vi "Finish.vi"   [LabVIEW 2014]
doc: "This VI is called just before exiting. It is expected to close I/O refnum, save collected data, etc."
uses:
  <vilib>/Rock Robotics/WPI/Joystick/WPI_JoystickGetSetRefNum.vi
  <vilib>/Rock Robotics/WPI/RobotDrive/WPI_RobotDriveGetSetRefNum.vi
  Robot Global Data.vi
  SimpleGyro/SimpleGyro.lvlib
types:
  T1 = typedef "WPI_MotorControlDeviceRef.ctl" = cluster{"DeviceStatus":errorcluster, "Type":T2, "PWM":cluster{"Controller":T3, "PWM Channel":T4, "DeadBand":T5}, "CAN":cluster{"Device Number":u8, "Control Mode":T6, "Semaphore":T7, "Max Vout":dbl, "TalonSRX Control Mode":T8}, "Invert":bool, "TransformRef":T9, "InvTransformRef":T9}
  T2 = typedef "WPI_MotorControlType.ctl" = enum16{"PWM", "CAN", "CANTalonSRX"}
  T3 = typedef "FPGA_TypedefDigitalModule.ctl" = enum16{"Controller 1"}
  T4 = typedef "FPGA_DIOPWMChannel.ctl" = enum8{"PWM 0", "PWM 1", "PWM 2", "PWM 3", "PWM 4", "PWM 5", "PWM 6", "PWM 7", "PWM 8", "PWM 9", "PWM MXP 0", "PWM MXP 1", "PWM MXP 2", "PWM MXP 3", "PWM MXP 4", "PWM MXP 5", "PWM MXP 6", "PWM MXP 7", "PWM MXP 8", "PWM MXP 9", "Invalid"}
  T5 = typedef "WPI_PWMDeadband.ctl" = cluster{"Name":string, "maxPositivePwm":i32, "minPositivePwm":i32, "centerPwm":i32, "maxNegativePwm":i32, "minNegativePwm":i32, "angularRange":u16}
  T6 = typedef "WPI_CANJaguar_ControlMode.ctl" = enum8{"Percent VBus", "Current", "Speed", "Position", "Voltage"}
  T7 = typedef "Semaphore RefNum" = refnum<k1>
  T8 = typedef "WPI_CANTalonSRX_APIControlMode.ctl" = enum8{"Percent VBus", "Speed", "Position", "Slave", "Unchanged / Invalid"}
  T9 = typedef "WPI_PWMTransform_ConPane.ctl" = refnum<vi>
  T10 = typedef "WPI_EncoderDevRef.ctl" = cluster{"DevStatus":errorcluster, "EncoderIndex":T11, "CounterIndex":T12, "DistancePerCount":dbl, "Decoding Type":T13}
  T11 = typedef "FPGA_EncoderIdx.ctl" = enum8{"Enc 0", "Enc 1", "Enc 2", "Enc 3", "Enc 4", "Enc 5", "Enc 6", "Enc 7", "Invalid"}
  T12 = typedef "FPGA_CounterCtrSystemIndex.ctl" = enum8{"Ctr 0", "Ctr 1", "Ctr 2", "Ctr 3", "Ctr 4", "Ctr 5", "Ctr 6", "Ctr 7", "Invalid"}
  T13 = typedef "WPI_EncoderType.ctl" = enum16{"1x", "2x", "4x"}
  T14 = typedef "WPI_I2CDevRef.ctl" = cluster{"DevStatus":errorcluster, "Controller":T3, "Device Address":u8, "Handle":i32, "I2C Bus":T15}
  T15 = typedef "i2c_bus.ctl" = enum16{"I2C On-Board", "I2C MXP", "Invalid"}
  T16 = typedef "WPI_RelayDevRef.ctl" = cluster{"DevStatus":errorcluster, "Relay Channel":T17, "Controller":T3, "Relay Direction":T18}
  T17 = typedef "FPGA_DIORelayChannel.ctl" = enum8{"Relay 0", "Relay 1", "Relay 2", "Relay 3", "Invalid"}
  T18 = typedef "WPI_RelayDirection.ctl" = enum16{"Both directions", "Forward only", "Reverse only"}
  T19 = typedef "WPI_JoystickDevRef.ctl" = cluster{"Device":T20}
  T20 = typedef "WPI_JoystickDeviceEnum.ctl" = enum16{"USB 0", "USB 1", "USB 2", "USB 3", "USB 4", "USB 5"}
  T21 = typedef "WPI_RobotDriveDevRef.ctl" = cluster{"DevStatus":errorcluster, "Motors[]":T1[], "Square Inputs":bool, "Max Output":dbl}
  T22 = typedef "SimpleGyro.lvlib/WPI_SimpleGyroDevRef.ctl" = cluster{"DevStatus":errorcluster, "Handle":i32, "Controller":T3, "SPI Bus":T23, "Device Found":bool, "Sample Rate":dbl}
  T23 = typedef "spi_bus.ctl" = enum16{"SPI On-Board, CS0", "SPI On-Board, CS1", "SPI On-Board, CS2", "SPI On-Board, CS3", "SPI MXP", "Invalid"}
  T24 = typedef "WPI_SwitchDevRef.ctl" = cluster{"DevStatus":errorcluster, "DIO Channel":T25, "Controller":T3, "CntIndex":T12, "Normally Closed":bool}
  T25 = typedef "FPGA_DIOChannel.ctl" = enum8{"DIO 0", "DIO 1", "DIO 2", "DIO 3", "DIO 4", "DIO 5", "DIO 6", "DIO 7", "DIO 8", "DIO 9", "DIO MXP 0", "DIO MXP 1", "DIO MXP 2", "DIO MXP 3", "DIO MXP 4", "DIO MXP 5", "DIO MXP 6", "DIO MXP 7", "DIO MXP 8", "DIO MXP 9", "DIO MXP 10", "DIO MXP 11", "DIO MXP 12", "DIO MXP 13", "DIO MXP 14", "DIO MXP 15", "Invalid"}
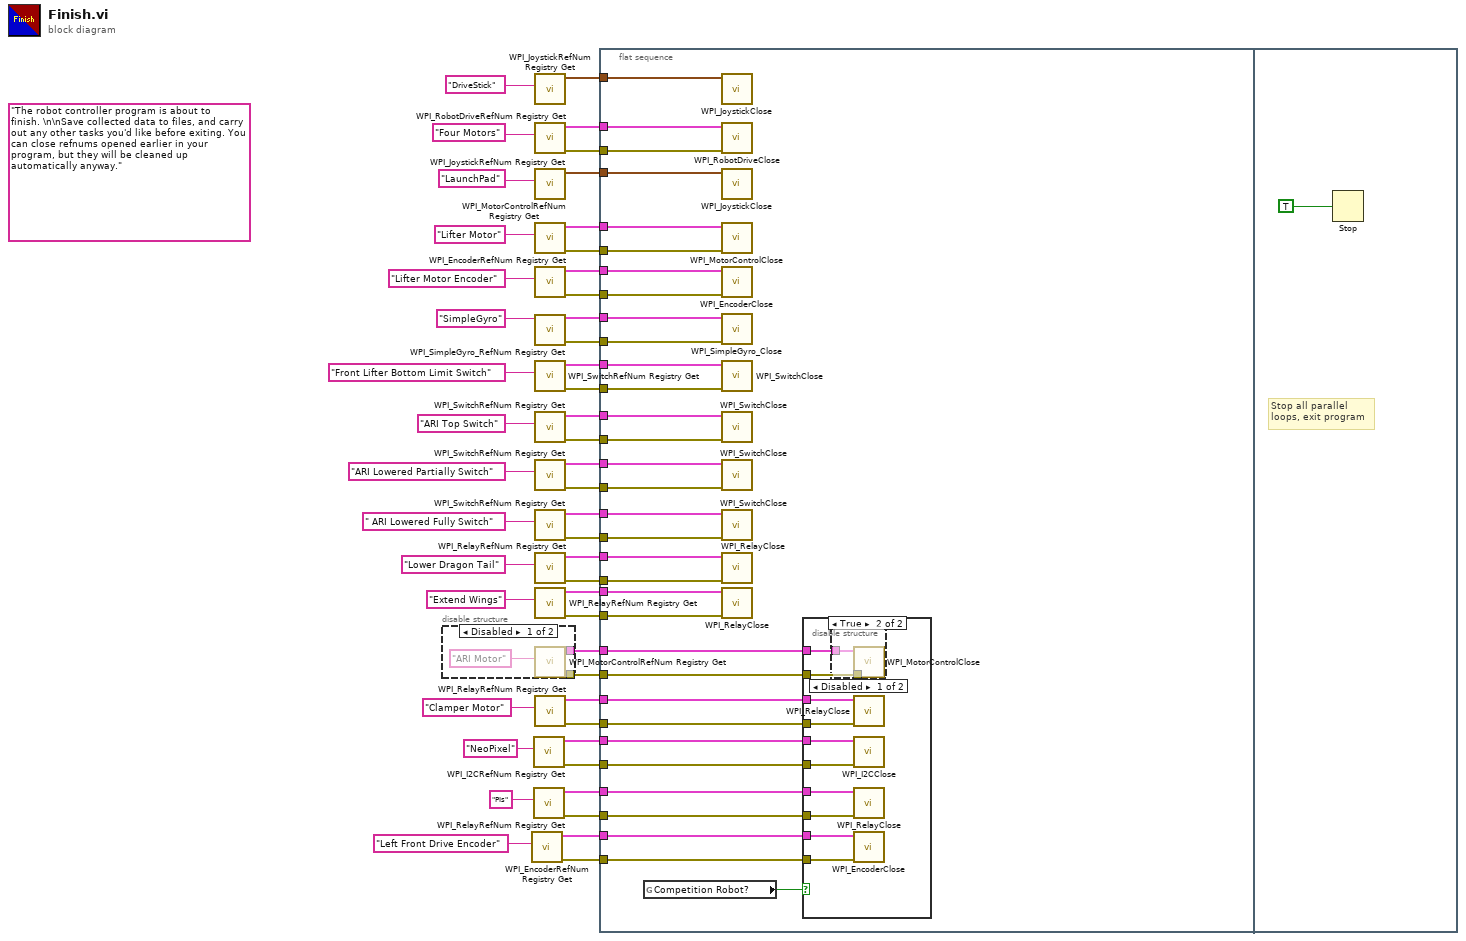
[diagram p0: block diagram]
diagram:
  (unwired) "The robot controller program is about to finish. \n\nSave collected data to files, and carry out any other tasks you'd like before exiting. You can close refnums opened earlier in your program, but they will be cleaned up automatically anyway."
  n1 = disable-structure shown="Disabled" {
    disable-tunnel: [w50 _] -> w19
    disable-tunnel: [w49 _] -> w18
    frame Disabled {
      n2 = call <vilib>:"WPI_MotorControlRefNum Registry Get.vi"("refnum name"="ARI Motor") -> ("error out"=w49:errorcluster, "MotorControlDevRef"=w50:T1)  [unwired: 9 in]
    }
    frame Enabled {
    }
  }
  n3 = call <vilib>:"WPI_EncoderRefNum Registry Get.vi"("refnum name"="Left Front Drive Encoder") -> ("error out"=w10:errorcluster, "EncoderDevRef"=w11:T10)  [unwired: 9 in]
  n4 = call <vilib>:"WPI_I2CRefNum Registry Get.vi"("refnum name"="NeoPixel") -> ("error out"=w14:errorcluster, "I2CDevRef"=w15:T14)  [unwired: 9 in]
  n5 = call <vilib>:"WPI_RelayRefNum Registry Get.vi"("refnum name"="PIs") -> ("error out"=w12:errorcluster, "RelayDevRef"=w13:T16)  [unwired: 9 in]
  n6 = call <vilib>:"WPI_JoystickRefNum Registry Get.vi"("refnum name"="DriveStick") -> ("JoystickDevRef"=w45:T19)  [unwired: 1 in, 9 out]
  n7 = call <vilib>:"WPI_RobotDriveRefNum Registry Get.vi"("refnum name"="Four Motors") -> ("error out"=w44:errorcluster, "RobotDriveDevRef"=w46:T21)  [unwired: 1 in, 8 out]
  n8 = call <vilib>:"WPI_JoystickRefNum Registry Get.vi"("refnum name"="LaunchPad") -> ("JoystickDevRef"=w42:T19)  [unwired: 1 in, 9 out]
  n9 = call <vilib>:"WPI_MotorControlRefNum Registry Get.vi"("refnum name"="Lifter Motor") -> ("error out"=w34:errorcluster, "MotorControlDevRef"=w35:T1)  [unwired: 9 in]
  n10 = call <vilib>:"WPI_EncoderRefNum Registry Get.vi"("refnum name"="Lifter Motor Encoder") -> ("error out"=w32:errorcluster, "EncoderDevRef"=w33:T10)  [unwired: 9 in]
  n11 = call "WPI_SimpleGyro_RefNum Registry Get.vi"("refnum name"="SimpleGyro") -> ("error out"=w7:errorcluster, "SimpleGyroDevRef"=w9:T22)  [unwired: 9 in]
  n12 = call <vilib>:"WPI_SwitchRefNum Registry Get.vi"("refnum name"="Front Lifter Bottom Limit Switch") -> ("error out"=w30:errorcluster, "SwitchDevRef"=w31:T24)  [unwired: 9 in]
  n13 = call <vilib>:"WPI_SwitchRefNum Registry Get.vi"("refnum name"="ARI Top Switch") -> ("error out"=w28:errorcluster, "SwitchDevRef"=w29:T24)  [unwired: 9 in]
  n14 = call <vilib>:"WPI_SwitchRefNum Registry Get.vi"("refnum name"="ARI Lowered Partially Switch") -> ("error out"=w26:errorcluster, "SwitchDevRef"=w27:T24)  [unwired: 9 in]
  n15 = call <vilib>:"WPI_SwitchRefNum Registry Get.vi"("refnum name"=" ARI Lowered Fully Switch") -> ("error out"=w24:errorcluster, "SwitchDevRef"=w25:T24)  [unwired: 9 in]
  n16 = call <vilib>:"WPI_RelayRefNum Registry Get.vi"("refnum name"="Lower Dragon Tail") -> ("error out"=w3:errorcluster, "RelayDevRef"=w4:T16)  [unwired: 9 in]
  n17 = call <vilib>:"WPI_RelayRefNum Registry Get.vi"("refnum name"="Extend Wings") -> ("error out"=w1:errorcluster, "RelayDevRef"=w2:T16)  [unwired: 9 in]
  n18 = call <vilib>:"WPI_RelayRefNum Registry Get.vi"("refnum name"="Clamper Motor") -> ("error out"=w16:errorcluster, "RelayDevRef"=w17:T16)  [unwired: 9 in]
  n19 = flat-sequence {
    tunnel: w46 -> [w84]
    tunnel: w45 -> [w83]
    tunnel: w44 -> [w82]
    tunnel: w42 -> [w81]
    tunnel: w35 -> [w80]
    tunnel: w34 -> [w79]
    tunnel: w33 -> [w78]
    tunnel: w32 -> [w77]
    tunnel: w31 -> [w76]
    tunnel: w30 -> [w75]
    tunnel: w29 -> [w74]
    tunnel: w28 -> [w73]
    tunnel: w27 -> [w72]
    tunnel: w26 -> [w71]
    tunnel: w25 -> [w70]
    tunnel: w24 -> [w69]
    tunnel: w19 -> [w68]
    tunnel: w18 -> [w67]
    tunnel: w17 -> [w66]
    tunnel: w16 -> [w65]
    tunnel: w15 -> [w64]
    tunnel: w14 -> [w63]
    tunnel: w13 -> [w62]
    tunnel: w12 -> [w61]
    tunnel: w11 -> [w60]
    tunnel: w10 -> [w59]
    tunnel: w9 -> [w58]
    tunnel: w7 -> [w57]
    tunnel: w4 -> [w55]
    tunnel: w3 -> [w54]
    tunnel: w2 -> [w53]
    tunnel: w1 -> [w52]
    frame #0 {
      n20 = global read "Robot Global Data.vi" "Competition Robot?"() -> (w56:bool)
      n21 = call <vilib>:"WPI_JoystickClose.vi"("JoystickDevRef"=w83) -> ()  [unwired: 11 out]
      n22 = call <vilib>:"WPI_RobotDriveClose.vi"("error in (no error)"=w82, "RobotDriveDevRef"=w84) -> ()  [unwired: 10 out]
      n23 = call <vilib>:"WPI_JoystickClose.vi"("JoystickDevRef"=w81) -> ()  [unwired: 11 out]
      n24 = call <vilib>:"WPI_MotorControlClose.vi"("error in (no error)"=w79, "MotorControlDevRef"=w80) -> ()  [unwired: 9 in, 1 out]
      n25 = call <vilib>:"WPI_EncoderClose.vi"("error in (no error)"=w77, "EncoderDevRef"=w78) -> ()  [unwired: 9 in, 1 out]
      n26 = call "WPI_SimpleGyro_Close.vi"("error in"=w57, "SimpleGyroDevRef"=w58) -> ()  [unwired: 9 in, 1 out]
      n27 = call <vilib>:"WPI_SwitchClose.vi"("error in (no error)"=w75, "SwitchDevRef"=w76) -> ()  [unwired: 9 in, 1 out]
      n28 = call <vilib>:"WPI_SwitchClose.vi"("error in (no error)"=w73, "SwitchDevRef"=w74) -> ()  [unwired: 9 in, 1 out]
      n29 = call <vilib>:"WPI_SwitchClose.vi"("error in (no error)"=w71, "SwitchDevRef"=w72) -> ()  [unwired: 9 in, 1 out]
      n30 = call <vilib>:"WPI_SwitchClose.vi"("error in (no error)"=w69, "SwitchDevRef"=w70) -> ()  [unwired: 9 in, 1 out]
      n31 = call <vilib>:"WPI_RelayClose.vi"("error in (no error)"=w54, "RelayDevRef"=w55) -> ()  [unwired: 9 in, 1 out]
      n32 = call <vilib>:"WPI_RelayClose.vi"("error in (no error)"=w52, "RelayDevRef"=w53) -> ()  [unwired: 9 in, 1 out]
      n33 = case shown="True" w56 {
        tunnel: w68 -> [_ w94]
        tunnel: w67 -> [_ w93]
        tunnel: w66 -> [_ w92]
        tunnel: w65 -> [_ w91]
        tunnel: w64 -> [_ w90]
        tunnel: w63 -> [_ w89]
        tunnel: w62 -> [_ w88]
        tunnel: w61 -> [_ w87]
        tunnel: w60 -> [_ w86]
        tunnel: w59 -> [_ w85]
        frame False {
        }
        frame True {
          n34 = disable-structure shown="Disabled" {
            disable-tunnel: w94 -> [w96 _]
            disable-tunnel: w93 -> [w95 _]
            frame Disabled {
              n35 = call <vilib>:"WPI_MotorControlClose.vi"("error in (no error)"=w95, "MotorControlDevRef"=w96) -> ()  [unwired: 9 in, 1 out]
            }
            frame Enabled {
            }
          }
          n36 = call <vilib>:"WPI_RelayClose.vi"("error in (no error)"=w91, "RelayDevRef"=w92) -> ()  [unwired: 9 in, 1 out]
          n37 = call <vilib>:"WPI_I2CClose.vi"("error in (no error)"=w89, "I2CDevRef"=w90) -> ()  [unwired: 9 in, 1 out]
          n38 = call <vilib>:"WPI_RelayClose.vi"("error in (no error)"=w87, "RelayDevRef"=w88) -> ()  [unwired: 9 in, 1 out]
          n39 = call <vilib>:"WPI_EncoderClose.vi"("error in (no error)"=w85, "EncoderDevRef"=w86) -> ()  [unwired: 9 in, 1 out]
        }
      }
    }
    frame #1 {
      # "Stop all parallel\nloops, exit program"
      n40 = Stop(stop? (T)=TRUE ("Quit")) -> ()
    }
  }
